vi "SDT_WriteFileDecayCurves.vi"(4 "SetUp[empty]":string, 5 "ActiveModule":string[](array[string]), 6 "EndTimeArray":dbl[](array[numeric]), 7 "DecayMatrix":u32[][](array[numeric]), 8 "ErrorIn":errorcluster, 9 "SPCdata":T13[](array[typedef]) {"scan_flyback" format="%x"}, 10 "FileType":T1=2 items=["non-Fifo"=1, "Fifo"=2, "FifoImage"=3], 11 "SDT-FilePath":path=path "\\\\lab13\\C/Users/jannis/Desktop/ZeissFifo.sdt") -> (0 "ErrorOut":errorcluster)   [LabVIEW 2017]
doc: "This VI writes a SDT-file to disc. The SetUp and the MeasureInfo blocks are created and appended with the data blocks. \nThis VI is limited to writing a DecayMatrix from a FIFO-Image recording and optional an IntensityImage to file. For single mode recordings use the spcmdll VI \\Public\\Configure\\Memory Transfer\\SPC_save_data_to_sdtfile.vi.\nFor a description of the format for the Data input cluster to this VI see the usage in \\Example\\ImagingEventStream-SimpleFifoImage.vi. Leave either of the cluster input arrays empty to not save them to disc.\nFor a description of the *.sdt file format see: SPC_data_file_structure.h\n\ninfo@becker-hickl.com"
uses:
  SPC_Wrappers/SPC_Controls/bhfile_header.ctl
  SPC_Wrappers/SPC_Controls/SPCdata.ctl
  SPC_Wrappers/SPC_Controls/MeasureInfo.ctl
  SPC_Wrappers/SPC_Controls/MeasureInfo_PartB.ctl
  SPC_Wrappers/SPC_Controls/MeasStopInfo.ctl
  SPC_Wrappers/SPC_Controls/MeasFCSInfo.ctl
  SPC_Wrappers/SPC_Controls/MeasureInfo_PartE.ctl
  SPC_Wrappers/SPC_Controls/MeasHISTInfo.ctl
  SPC_Wrappers/SPC_Controls/HISTInfoExt.ctl
  SPC_Wrappers/SPC_Controls/MeasureInfo_PartI.ctl
  SPC_Wrappers/SPC_Controls/MeasureInfo_PartK.ctl
  SPC_Wrappers/SPC_Controls/MeasureInfo_PartM.ctl
  SPC_Wrappers/SPC_Controls/BHFileBlockHeader.ctl
  SPC_Wrappers/SPC_Controls/FileType.ctl
  SDT_CreateModTypeString.vi
  SDT_MeasureBlockToString.vi
panel:
  out "Info Block":string
  out "BHFileBlockHeaders":T2[](array[typedef])
  out "MeasureInfos":T3[](array[typedef]) {"MeasFCSInfo"."end_time" format="%#_7g"; "MeasStopInfo"."flags" format="x%x"}
  out "BlockLengths":i32[](array[numeric])
  out "bhfile_header":T14 {"chksum" format="x%x"; "header_valid" format="x%x"}
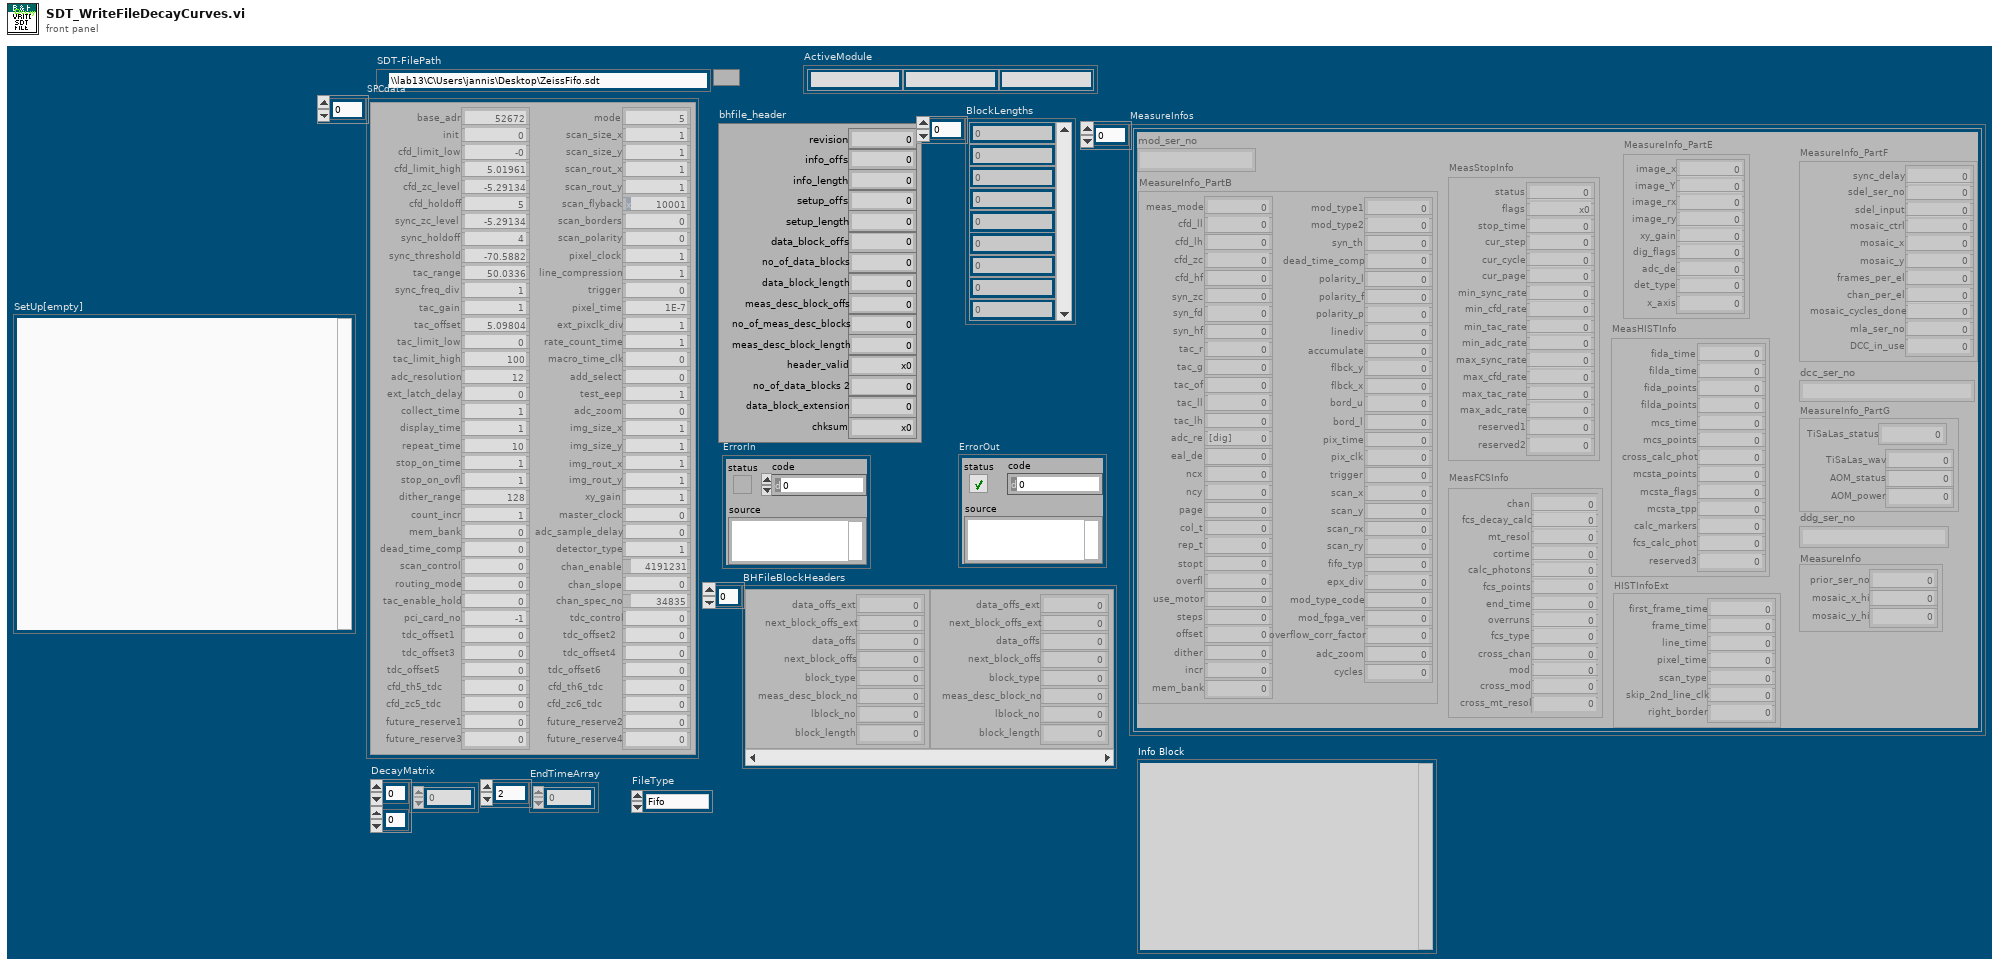
[diagram p1: front panel]
types:
  T1 = typedef "FileType.ctl" = u16
  T2 = typedef "BHFileBlockHeader.ctl" = cluster{"data_offs_ext":u8, "next_block_offs_ext":u8, "data_offs":u32, "next_block_offs":u32, "block_type":u16, "meas_desc_block_no":i16, "lblock_no":u32, "block_length":u32}
  T3 = typedef "MeasureInfo.ctl" = cluster{"mod_ser_no":string, "MeasureInfo_PartB":T4, "MeasStopInfo":T5, "MeasFCSInfo":T6, "MeasureInfo_PartE":T7, "MeasHISTInfo":T8, "HISTInfoExt":T9, "MeasureInfo_PartF":T10, "dcc_ser_no":string, "MeasureInfo_PartG":T11, "ddg_ser_no":string, "MeasureInfo":T12}
  T4 = typedef "MeasureInfo_PartB.ctl" = cluster{"meas_mode":i16, "cfd_ll":sgl, "cfd_lh":sgl, "cfd_zc":sgl, "cfd_hf":sgl, "syn_zc":sgl, "syn_fd":i16, "syn_hf":sgl, "tac_r":sgl, "tac_g":i16, "tac_of":sgl, "tac_ll":sgl, "tac_lh":sgl, "adc_re":i16, "eal_de":i16, "ncx":i16, "ncy":i16, "page":u16, "col_t":sgl, "rep_t":sgl, "stopt":i16, "overfl":i8, "use_motor":i16, "steps":u16, "offset":sgl, "dither":i16, "incr":i16, "mem_bank":i16, "mod_type1":u64, "mod_type2":u64, "syn_th":sgl, "dead_time_comp":i16, "polarity_l":i16, "polarity_f":i16, "polarity_p":i16, "linediv":i16, "accumulate":i16, "flbck_y":i32, "flbck_x":i32, "bord_u":i32, "bord_l":i32, "pix_time":sgl, "pix_clk":i16, "trigger":i16, "scan_x":i32, "scan_y":i32, "scan_rx":i32, "scan_ry":i32, "fifo_typ":i16, "epx_div":i32, "mod_type_code":u16, "mod_fpga_ver":u16, "overflow_corr_factor":sgl, "adc_zoom":i32, "cycles":i32}
  T5 = typedef "MeasStopInfo.ctl" = cluster{"status":u16, "flags":u16, "stop_time":sgl, "cur_step":i32, "cur_cycle":i32, "cur_page":i32, "min_sync_rate":sgl, "min_cfd_rate":sgl, "min_tac_rate":sgl, "min_adc_rate":sgl, "max_sync_rate":sgl, "max_cfd_rate":sgl, "max_tac_rate":sgl, "max_adc_rate":sgl, "reserved1":i32, "reserved2":sgl}
  T6 = typedef "MeasFCSInfo.ctl" = cluster{"chan":u16, "fcs_decay_calc":u16, "mt_resol":u32, "cortime":sgl, "calc_photons":u32, "fcs_points":i32, "end_time":sgl, "overruns":u16, "fcs_type":u16, "cross_chan":u16, "mod":u16, "cross_mod":u16, "cross_mt_resol":u32}
  T7 = typedef "MeasureInfo_PartE.ctl" = cluster{"image_x":i32, "image_Y":i32, "image_rx":i32, "image_ry":i32, "xy_gain":i16, "dig_flags":i16, "adc_de":i16, "det_type":i16, "x_axis":i16}
  T8 = typedef "MeasHISTInfo.ctl" = cluster{"fida_time":sgl, "filda_time":sgl, "fida_points":i32, "filda_points":i32, "mcs_time":sgl, "mcs_points":i32, "cross_calc_phot":u32, "mcsta_points":u16, "mcsta_flags":u16, "mcsta_tpp":u32, "calc_markers":u32, "fcs_calc_phot":u32, "reserved3":u32}
  T9 = typedef "HISTInfoExt.ctl" = cluster{"first_frame_time":sgl, "frame_time":sgl, "line_time":sgl, "pixel_time":sgl, "scan_type":i16, "skip_2nd_line_clk":i16, "right_border":u32}
  T10 = typedef "MeasureInfo_PartI.ctl" = cluster{"sync_delay":sgl, "sdel_ser_no":u16, "sdel_input":i8, "mosaic_ctrl":i8, "mosaic_x":u8, "mosaic_y":u8, "frames_per_el":i16, "chan_per_el":i16, "mosaic_cycles_done":i32, "mla_ser_no":u16, "DCC_in_use":u8}
  T11 = typedef "MeasureInfo_PartK.ctl" = cluster{"TiSaLas_status":u16, "TiSaLas_wav":u16, "AOM_status":u8, "AOM_power":u8}
  T12 = typedef "MeasureInfo_PartM.ctl" = cluster{"prior_ser_no":i32, "mosaic_x_hi":u8, "mosaic_y_hi":u8}
  T13 = typedef "SPCdata.ctl" = cluster{"base_adr":u16, "init":i16, "cfd_limit_low":sgl, "cfd_limit_high":sgl, "cfd_zc_level":sgl, "cfd_holdoff":sgl, "sync_zc_level":sgl, "sync_holdoff":sgl, "sync_threshold":sgl, "tac_range":sgl, "sync_freq_div":i16, "tac_gain":i16, "tac_offset":sgl, "tac_limit_low":sgl, "tac_limit_high":sgl, "adc_resolution":i16, "ext_latch_delay":i16, "collect_time":sgl, "display_time":sgl, "repeat_time":sgl, "stop_on_time":i16, "stop_on_ovfl":i16, "dither_range":i16, "count_incr":i16, "mem_bank":i16, "dead_time_comp":i16, "scan_control":u16, "routing_mode":u16, "tac_enable_hold":sgl, "pci_card_no":i16, "mode":u16, "scan_size_x":u32, "scan_size_y":u32, "scan_rout_x":u32, "scan_rout_y":u32, "scan_flyback":u32, "scan_borders":u32, "scan_polarity":u16, "pixel_clock":u16, "line_compression":u16, "trigger":u16, "pixel_time":sgl, "ext_pixclk_div":u32, "rate_count_time":sgl, "macro_time_clk":i16, "add_select":i16, "test_eep":i16, "adc_zoom":i16, "img_size_x":u32, "img_size_y":u32, "img_rout_x":u32, "img_rout_y":u32, "xy_gain":i16, "master_clock":i16, "adc_sample_delay":i16, "detector_type":i16, "chan_enable":u32, "chan_slope":u32, "chan_spec_no":u32, "tdc_control":u32, "tdc_offset1":sgl, "tdc_offset2":sgl, "tdc_offset3":sgl, "tdc_offset4":sgl, "tdc_offset5":sgl, "tdc_offset6":sgl, "cfd_th5_tdc":sgl, "cfd_th6_tdc":sgl, "cfd_zc5_tdc":sgl, "cfd_zc6_tdc":sgl, "future_reserve1":u64, "future_reserve2":u64, "future_reserve3":u64, "future_reserve4":u64}
  T14 = typedef "bhfile_header.ctl" = cluster{"revision":i16, "info_offs":i32, "info_length":i16, "setup_offs":i32, "setup_length":u16, "data_block_offs":i32, "no_of_data_blocks":i16, "data_block_length":u32, "meas_desc_block_offs":i32, "no_of_meas_desc_blocks":i16, "meas_desc_block_length":i16, "header_valid":u16, "no_of_data_blocks 2":u32, "data_block_extension":u16, "chksum":u16}
  T15 = enum16{"open", "replace", "create", "open or create", "replace or create", "replace or create with confirmation"}
  T16 = enum16{"big-endian, network order", "native, host order", "little-endian"}
  T17 = typedef "BHModuleType.ctl" = i16
  T18 = typedef "ModuleType.ctl" = i16
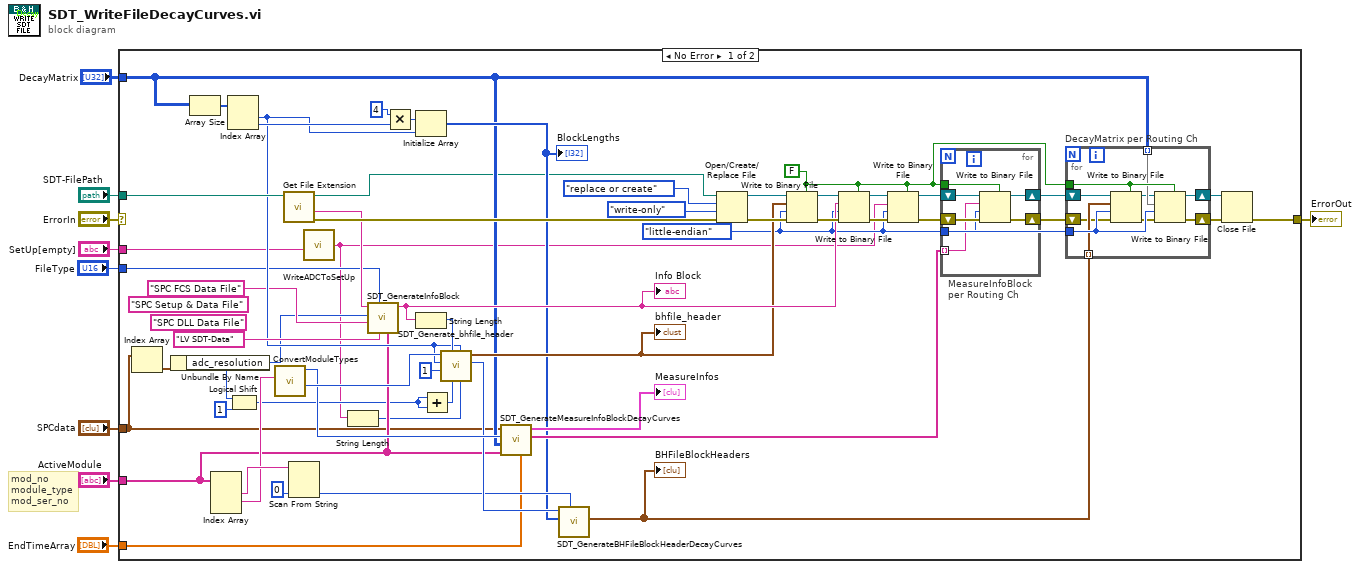
[diagram p0: block diagram]
diagram:
  # "mod_no\nmodule_type\nmod_ser_no"
  n1 = case shown="No Error" "ErrorIn" {
    selector: "ErrorIn" -> [_ w83]
    tunnel: [w10 w83] -> w8
    tunnel: "SPCdata" -> [w16 _]
    tunnel: "ActiveModule" -> [w25 _]
    tunnel: "SDT-FilePath" -> [w38 _]
    tunnel: "DecayMatrix" -> [w35 _]
    tunnel: "EndTimeArray" -> [w28 _]
    tunnel: "FileType" -> [w27 _]
    tunnel: "SetUp[empty]" -> [w12 _]
    frame No Error {
      (unwired) "SPC Setup & Data File" ("FileID")
      (unwired) "SPC DLL Data File" ("FileID")
      w20 = FALSE ("prepend array or string size? (T)")
      w19 = T16."little-endian" ("byte order (0:big-endian, network order)")
      n2 = Index Array(array=w16) -> (element=w17:T13)  [unwired: 1 in]
      n3 = Unbundle By Name(w17) -> ("adc_resolution"=w14:i16)
      n4 = Array Size(array=w35) -> (size(s)=w52:i32[])
      n5 = Index Array(array=w25) -> (element #1=w56:string, element #2=w53:string)  [unwired: 3 in, 1 out]
      n6 = Index Array(array=w52) -> (element #1=w32:i32, element #2=w34:i32)  [unwired: 2 in]
      n7 = Logical Shift(y=w14, x=u32 1) -> (x << y=w13:u32)
      n8 = call "ConvertModuleTypes.vi"("ModuleTypeStringIn"=w53) -> ("BHModuleType"=w45:T17, "Module TypeOut"=w44:T18)  [unwired: 8 in, 1 out]
      n9 = call <vilib>:"Get File Extension.vi"("file"=w38) -> ("error out"=w61:errorcluster, "filename without extension"=w49:string, "dup file"=w26:path)  [unwired: 6 in, 2 out]
      n10 = Scan From String(input string=w56, default 1=u32 0 ("meas_desc_block_no")) -> (output 1=w39:u32)  [unwired: 3 in, 3 out]
      n11 = call "WriteADCToSetUp.vi"("ASCIISetUp"=w12) -> ("ASCIISetUpOut"=w11:string)  [unwired: 6 in]
      n12 = String Length(string=w11) -> (length=w18:i32)
      n13 = call "SDT_GenerateInfoBlock.vi"("ActiveModule"=w25, "Contents"="LV SDT-Data", "FileType"=w27, "FileID"="SPC FCS Data File", "adc_re[exp]"=w14, "FilenameNoExtension"=w49) -> ("Info Block"=w47:string)  [unwired: 5 in]
      "Info Block" <- w47
      n14 = Multiply(x=4 ("y"), y=w34) -> (x*y=w33:i32)
      n15 = Initialize Array(w33, w32) -> (w36:i32[])
      "BlockLengths" <- w36
      n16 = String Length(string=w47) -> (length=w46:i32)
      n17 = Add(x=w13, y=w13) -> (x+y=w30:u32)
      n18 = call "SDT_Generate_bhfile_header.vi"("setup_length"=w18, "no_of_data_blocks"=w32, "adc_re[dig]"=w30, "info_length"=w46, "ImageSize"=u32 1, "NoOfRoutingChannel"=w32, "BHModuleType"=w45) -> ("data_block_offs"=w40:i32, "bhfile_header"=w42:T14)  [unwired: 3 in]
      "bhfile_header" <- w42
      n19 = call "SDT_GenerateMeasureInfoBlockDecayCurves.vi"("EndTimeArray"=w28, "ActiveModule"=w25, "DecayMatrix"=w35, "Module Type"=w44, "SPCdata"=w16) -> ("MeasureInfoStrings"=w37:string[], "MeasureInfos"=→"MeasureInfos":T3[])  [unwired: 5 in]
      n20 = call "SDT_GenerateBHFileBlockHeaderDecayCurves.vi"("ModuleNo"=w39, "BlockLengths"=w36, "data_block_offs"=w40) -> ("BHFileBlockHeaders"=w41:T2[])  [unwired: 7 in, 1 out]
      "BHFileBlockHeaders" <- w41
      n21 = Open/Create/Replace File(file path (use dialog)=w26, error in=w61, operation (0:open)=T15."replace or create", access (0:read/write)=enum16{"read/write", "read-only", "write-only"}."write-only") -> (refnum out=w63:refnum<file>, error out=w60:errorcluster)  [unwired: 2 in, 1 out]
      n22 = Write to Binary File(file (use dialog)=w63, data=w42, error in=w60, 5:w20, 9:w19) -> (refnum out=w62:refnum<file>, error out=w59:errorcluster)  [unwired: 1 in, 1 out]
      n23 = Write to Binary File(file (use dialog)=w62, data=w47, error in=w59, 5:w20, 9:w19) -> (refnum out=w22:refnum<file>, error out=w24:errorcluster)  [unwired: 1 in, 1 out]
      n24 = Write to Binary File(file (use dialog)=w22, data=w11, error in=w24, 5:w20, 9:w19) -> (refnum out=w21:refnum<file>, error out=w23:errorcluster)  [unwired: 1 in, 1 out]
      n25 = for "MeasureInfoBlock\nper Routing Ch" {
        tunnel: w20 -> [w70]
        tunnel: w19 -> [w69]
        shift-right: [w68] -> w51
        shift-left: w21 -> [w72]
        shift-right: [w67] -> w50
        shift-left: w23 -> [w71]
        tunnel: w37 -> [w66] mode=indexing
        n26 = Write to Binary File(file (use dialog)=w72, data=w66, error in=w71, 5:w70, 9:w69) -> (refnum out=w68:refnum<file>, error out=w67:errorcluster)  [unwired: 1 in, 1 out]
      }
      n27 = for "DecayMatrix per Routing Ch" {
        tunnel: w20 -> [w82]
        tunnel: w19 -> [w81]
        tunnel: w41 -> [w78] mode=indexing
        tunnel: w35 -> [w77] mode=indexing
        shift-right: [w79] -> w57
        shift-left: w51 -> [w76]
        shift-right: [w80] -> w58
        shift-left: w50 -> [w75]
        n28 = Write to Binary File(file (use dialog)=w76, data=w78, error in=w75, 5:w82, 9:w81) -> (refnum out=w74:refnum<file>, error out=w73:errorcluster)  [unwired: 1 in, 1 out]
        n29 = Write to Binary File(file (use dialog)=w74, data=w77, error in=w73, 5:w82, 9:w81) -> (refnum out=w79:refnum<file>, error out=w80:errorcluster)  [unwired: 1 in, 1 out]
      }
      n30 = Close File(refnum=w57, error in=w58) -> (error out=w10:errorcluster)  [unwired: 1 out]
    }
    frame Error {
    }
  }
  "ErrorOut" <- w8
